vi "setOdoConf.vi"(7 "axisStr":string, 8 "error in (no error)":errorcluster, 11 "pHandle":u32) -> (0 "error out":errorcluster, 3 "return type":i32)   [LabVIEW 2011, in "sbgLabView.lvlib"]
uses:
  sbgLabView.lvlib
  sbgMatLab.dll
panel:
  in  "gpsGainCorrection":bool
  in  "gainError":u8
  in  "pulsesPerMeter":sgl
  in  "channel":u8
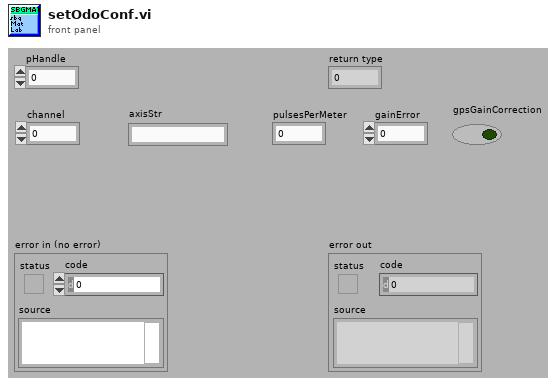
[diagram p1: front panel]
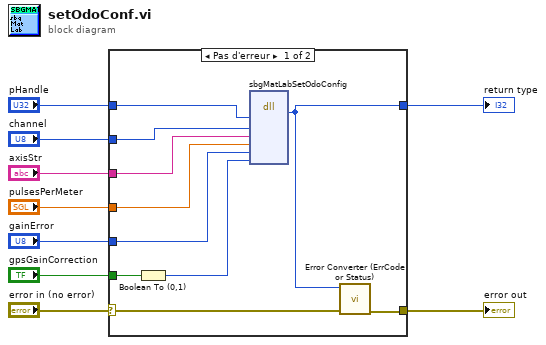
[diagram p0: block diagram]
diagram:
  n1 = case shown="Pas d'erreur" "error in (no error)" {
    selector: "error in (no error)" -> [w17 w20]
    tunnel: [w16 w20] -> w8
    tunnel: [w19 _] -> w7
    tunnel: "pHandle" -> [w18 _]
    tunnel: "axisStr" -> [w14 _]
    tunnel: "channel" -> [w15 _]
    tunnel: "pulsesPerMeter" -> [w13 _]
    tunnel: "gainError" -> [w12 _]
    tunnel: "gpsGainCorrection" -> [w11 _]
    frame No Error {
      n2 = Boolean To (0,1)(Boolean=w11) -> (0, 1=w10:i16)
      n3 = dll-call lib="C:/SBG-Systems/remote/projects/software/projects/labviewExample/sbgLabView/sbgMatLab.*" fn="sbgMatLabSetOdoConfig" ("sbgMatLab.dll:sbgMatLabSetGpsOptions")("pHandle"=w18, "channel"=w15, "axisStr"=w14, "pulsesPerMeter"=w13, "gainError"=w12, "gpsGainCorrection"=w10) -> ("return type"=w19:i32)  [unwired: 9 in, 2 out]
      n4 = call "Error Converter (ErrCode or Status).vi"("error in (no error)"=w17, "error code"=w19) -> ("error out"=w16:errorcluster)  [unwired: 9 in]
    }
    frame Error {
    }
  }
  "return type" <- w7
  "error out" <- w8
